vi "interOpTest.vi"(11 "input":dbl) -> (3 "output":dbl)   [LabVIEW 2016]
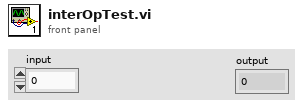
[diagram p1: front panel]
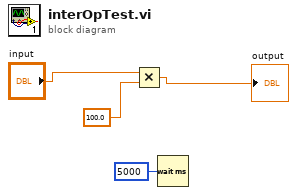
[diagram p0: block diagram]
diagram:
  n1 = Multiply(x="input", y=100.0) -> (x*y=→"output":dbl)
  n2 = Wait (ms)(milliseconds to wait=u32 5000) -> ()  [unwired: 1 out]
